vi "3-1.vi"() -> ()   [LabVIEW 2014]
panel:
  out "?":string
  out "Warning?":bool
  in  "Min Temp.":dbl
  in  "Max Temp.":dbl
  in  "Current Temp.":dbl
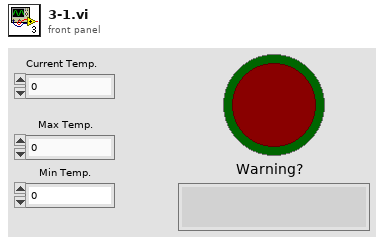
[diagram p1: front panel]
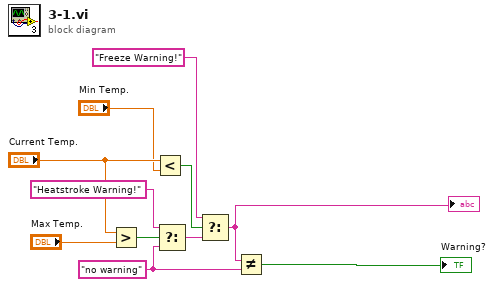
[diagram p0: block diagram]
diagram:
  w11 = "no warning"
  n1 = Greater?(x="Current Temp.", y="Max Temp.") -> (0:w4:bool)
  n2 = Less?(x="Current Temp.", y="Min Temp.") -> (x < y?=w1:bool)
  n3 = Select(t="Heatstroke Warning!", s=w4, f=w11) -> (s? t:f=w6:string)
  n4 = Select(t="Freeze Warning!", s=w1, f=w6) -> (s? t:f=w7:string)
  "?" <- w7
  n5 = Not Equal?(x=w7, y=w11) -> (x != y?=→"Warning?":bool)
